vi "G#Object_ErrorMissingMethod.vi"(0 "reference in":refnum<class "IG#.lvclass">, 5 "error in (no error)":errorcluster, 7 "call depth (1)":i32=1) -> (14 "reference out":refnum<class "IG#.lvclass">, 19 "error out":errorcluster)   [LabVIEW 2020, in "IG#.lvclass"]
doc: "Sets an error to indicate that a abstract method is not implemented."
uses:
  <vilib>/addons/_AddQ/IG#/IG#.lvclass
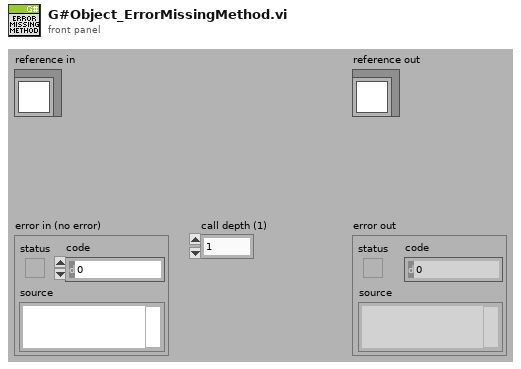
[diagram p1: front panel]
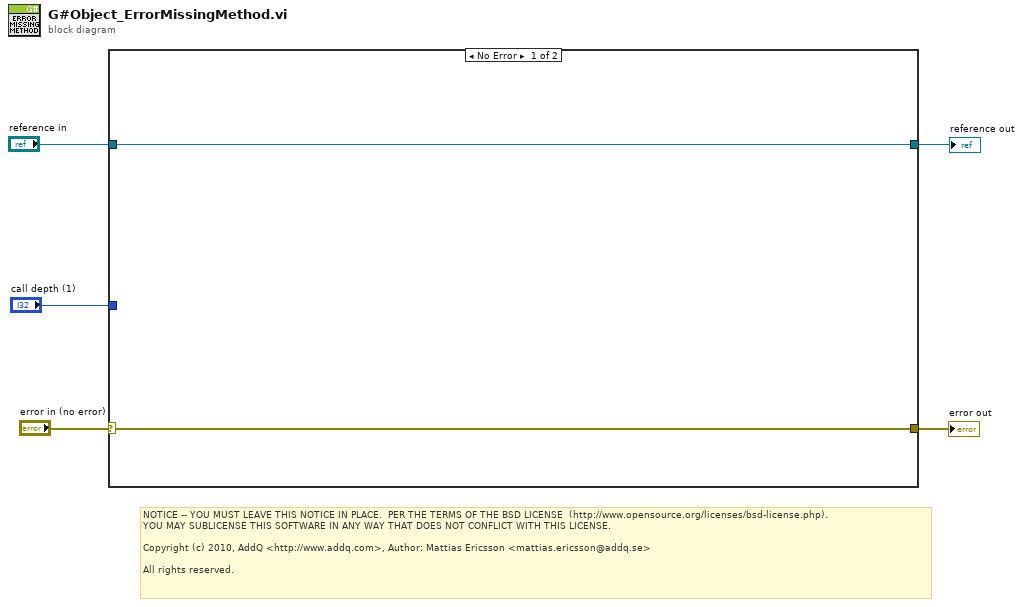
[diagram p0: block diagram]
diagram:
  # "NOTICE -- YOU MUST LEAVE THIS NOTICE IN PLACE.  PER THE TERMS OF THE BSD LICENSE  (http://www.opensource.org/licenses/bsd-license.php).\nYOU MAY SUBLICENSE THIS SOFTWARE IN ANY WAY THAT DOES NOT CONFLICT WITH THIS LICENSE.\n\nCopyright (c) 2010, AddQ <http://www.addq.com>, Author: Mattias Ericsson <mattias.ericsson@addq.se>\n\nAll rights reserved."
  n1 = case shown="No Error" "error in (no error)" {
    selector: "error in (no error)" -> [w6 w9]
    tunnel: [w6 w9] -> w1
    tunnel: "call depth (1)" -> [_ _]
    tunnel: "reference in" -> [w7 w8]
    tunnel: [w7 w8] -> w3
    frame No Error {
    }
    frame Error {
    }
  }
  "reference out" <- w3
  "error out" <- w1
